vi "Parse Node.vi"(7 "Parent ID":string, 8 "error in (no error)":errorcluster, 10 "Node in":refnum<k20>, 11 "Tree in":refnum<data-value>) -> (0 "error out":errorcluster, 2 "Node out":refnum<k20>, 3 "Tree out":refnum<data-value>, 5 "Unique ID":string)   [LabVIEW 2016]
uses:
  <vilib>/ni/Tree/Tree Manager/Tree.lvclass
  <vilib>/ni/Tree/Data Types/String/String.lvclass/String.ctl
  <vilib>/ni/Tree/Data Types/String/To String Tree Data.vi
  <vilib>/ni/Tree/Data Types/String/String.lvclass
  C:/Program Files/National Instruments/LabVIEW 2016/vi.lib/ni/Tree/Tree Data/Tree Data.lvclass
  <vilib>/ni/Tree/Tree Manager/API/Set Attributes Tree Data.vi
  <vilib>/ni/Tree/Tree Manager/API/Set Meta Data.vi
  <resource>/objmgr/DOMUserDefRef.rc
  <vilib>/xml/NI_XML.lvlib
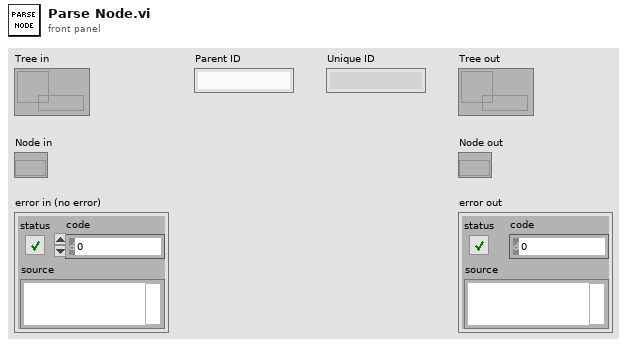
[diagram p1: front panel]
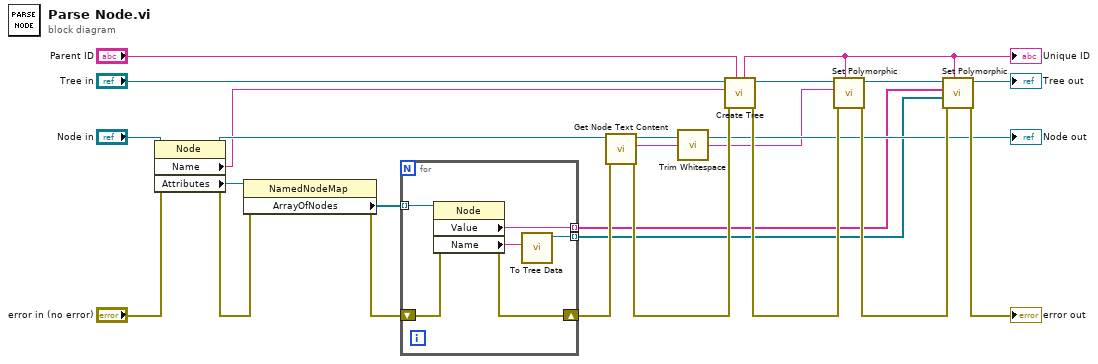
[diagram p0: block diagram]
diagram:
  n1 = property class="Node"(reference="Node in", error in="error in (no error)") -> (reference out=w11:refnum<k20>, error out=w21:errorcluster, "Name"=w5:string, "Attributes"=w3:refnum<k20>)
  n2 = property class="NamedNodeMap"(reference=w3, error in=w21) -> (error out=w22:errorcluster, "ArrayOfNodes"=w4:refnum<k20>[])  [unwired: 1 out]
  n3 = for {
    tunnel: w4 -> [w28] mode=indexing
    shift-right: [w29] -> w18
    shift-left: w22 -> [w30]
    tunnel: [w25] -> w8 mode=indexing
    tunnel: [w26] -> w7 mode=indexing
    n4 = property class="Node"(reference=w28, error in=w30) -> (error out=w29:errorcluster, "Value"=w26:string, "Name"=w27:string)  [unwired: 1 out]
    n5 = call-poly <vilib>:"To Tree Data.vi"("String"=w27) -> ("String Tree Data"=w25:refnum<class "String.lvclass">)  [unwired: 10 in]
  }
  n6 = call <vilib>:"Get Node Text Content.vi"("error in (no error)"=w18, "node in"=w11) -> ("error out"=w19:errorcluster, "node text"=w16:string, "node out"=→"Node out":refnum<k20>)  [unwired: 7 in]
  n7 = call <vilib>:"Trim Whitespace.vi"("string"=w16) -> ("trimmed string"=w1:string)  [unwired: 1 in]
  n8 = call <vilib>:"Create Tree.vi"("Parent ID (empty)"="Parent ID", "Error In"=w19, "Name"=w5, "Tree Manager"="Tree in") -> ("Error Out"=w23:errorcluster, "Tree Manager"=w6:refnum<data-value>, "Unique ID"=w15:string)  [unwired: 5 in]
  "Unique ID" <- w15
  n9 = call-poly <vilib>:"Set Polymorphic.vi"("Tree ID"=w15, "Error In"=w23, "Meta Data"=w1, "Tree Manager"=w6) -> ("Error Out"=w24:errorcluster, "Tree Manager"=w14:refnum<data-value>)  [unwired: 6 in]
  n10 = call-poly <vilib>:"Set Polymorphic.vi"("Tree ID"=w15, "Error In"=w24, "Attributes Values"=w8, "Attributes Names"=w7, "Tree Manager"=w14) -> ("Error Out"=→"error out":errorcluster, "Tree Manager"=→"Tree out":refnum<data-value>)  [unwired: 4 in, 1 out]
